vi "TX_POWER(DEBUG).vi"() -> ()   [LabVIEW 2015]
uses:
  <instrlib>/Rohde&Schwarz Spectrum Analyzer/Rohde&Schwarz Spectrum Analyzer.lvlib
panel:
  in  "O_R&S Spec1 2":refnum<visa-resource-name>
  in  "O_R&S Spec1":refnum<visa-resource-name>="GPIB0::22::INSTR"
  out "R_B_peak":dbl[](array[numeric])
  out "R_B_pos":dbl[](array[numeric])
  out "R_A_peak":dbl[](array[numeric])
  out "R_A_pos":dbl[](array[numeric])
  out "B通道接收带":cluster{"X":dbl[], "Amplitude":dbl[]}(graph)
  out "B通道发射带":cluster{"X":dbl[], "Amplitude":dbl[]}(graph)
  out "A通道发射带":cluster{"X":dbl[], "Amplitude":dbl[]}(graph)
  out "A通道接收带":cluster{"X":dbl[], "Amplitude":dbl[]}(graph)
  in  "接收带末频率(Mhz)":u32=2300 caption="Start Frequency (0.0)"
  in  "接收带始频率(Mhz)":u32=2200 caption="Stop Frequency (0.0)"
  out "R_B_paek":dbl caption="Marker Amplitude" format="%^.3e"
  out "R_B_pos":dbl caption="Marker Position" format="%^.3e"
  out "Amplitude 2":dbl[](array[numeric]) caption="Amplitude" format="%^.3e"
  out "X 2":dbl[](array[numeric]) caption="X" format="%^.3e"
  out "R_A_peak":dbl caption="Marker Amplitude" format="%^.3e"
  out "R_A_pos":dbl caption="Marker Position" format="%^.3e"
  out "Amplitude":dbl[](array[numeric]) format="%^.3e"
  out "X":dbl[](array[numeric]) format="%^.3e"
  in  "发射带末频率(Mhz)":u32=2130 caption="Start Frequency (0.0)"
  in  "发射带始频率(Mhz)":u32=2018 caption="Stop Frequency (0.0)"
  out "B_peak":dbl[](array[numeric])
  out "B_pos":dbl[](array[numeric])
  out "B_next_pos":dbl[](array[numeric])
  out "B_peak_next":dbl[](array[numeric])
  out "Array 6":cluster{"X":dbl[], "Amplitude":dbl[]}[](array[cluster])
  out "A_peak":dbl[](array[numeric])
  out "A_pos":dbl[](array[numeric])
  out "A_next_pos":dbl[](array[numeric])
  out "A_peak_next":dbl[](array[numeric])
  out "Array":cluster{"X":dbl[], "Amplitude":dbl[]}[](array[cluster])
  in  "OK":bool
  in  "stop":bool
  out "Bx":dbl[](array[numeric]) caption="X" format="%^.3e"
  out "By":dbl[](array[numeric]) caption="Amplitude" format="%^.3e"
  out "B_pos":dbl caption="Marker Position" format="%^.3e"
  out "B_peak":dbl caption="Marker Amplitude" format="%^.3e"
  out "B_next_pos":dbl caption="Marker Position" format="%^.3e"
  out "B_peak_next":dbl caption="Marker Amplitude" format="%^.3e"
  out "A_peak_next":dbl caption="Marker Amplitude" format="%^.3e"
  out "A_next_pos":dbl caption="Marker Position" format="%^.3e"
  out "A_peak":dbl caption="Marker Amplitude" format="%^.3e"
  out "A_pos":dbl caption="Marker Position" format="%^.3e"
  out "Ay":dbl[](array[numeric]) caption="Amplitude" format="%^.3e"
  out "Ax":dbl[](array[numeric]) caption="X" format="%^.3e"
  in  "VISA resource name 2":refnum<visa-resource-name>="COM3"
  out "Freq_Tab":u32[](array[numeric])
  in  "Insert Point":u32
  in  "EABLE Insert":bool
  in  "Value":u32=10 caption="Point Num"
  in  "cnt/setp":enum16{"SETP", "COUNT"}(ring)=enum."COUNT"
  in  "freq_max(Mhz)":u32=2123
  in  "freq_min(Mhz)":u32=2018
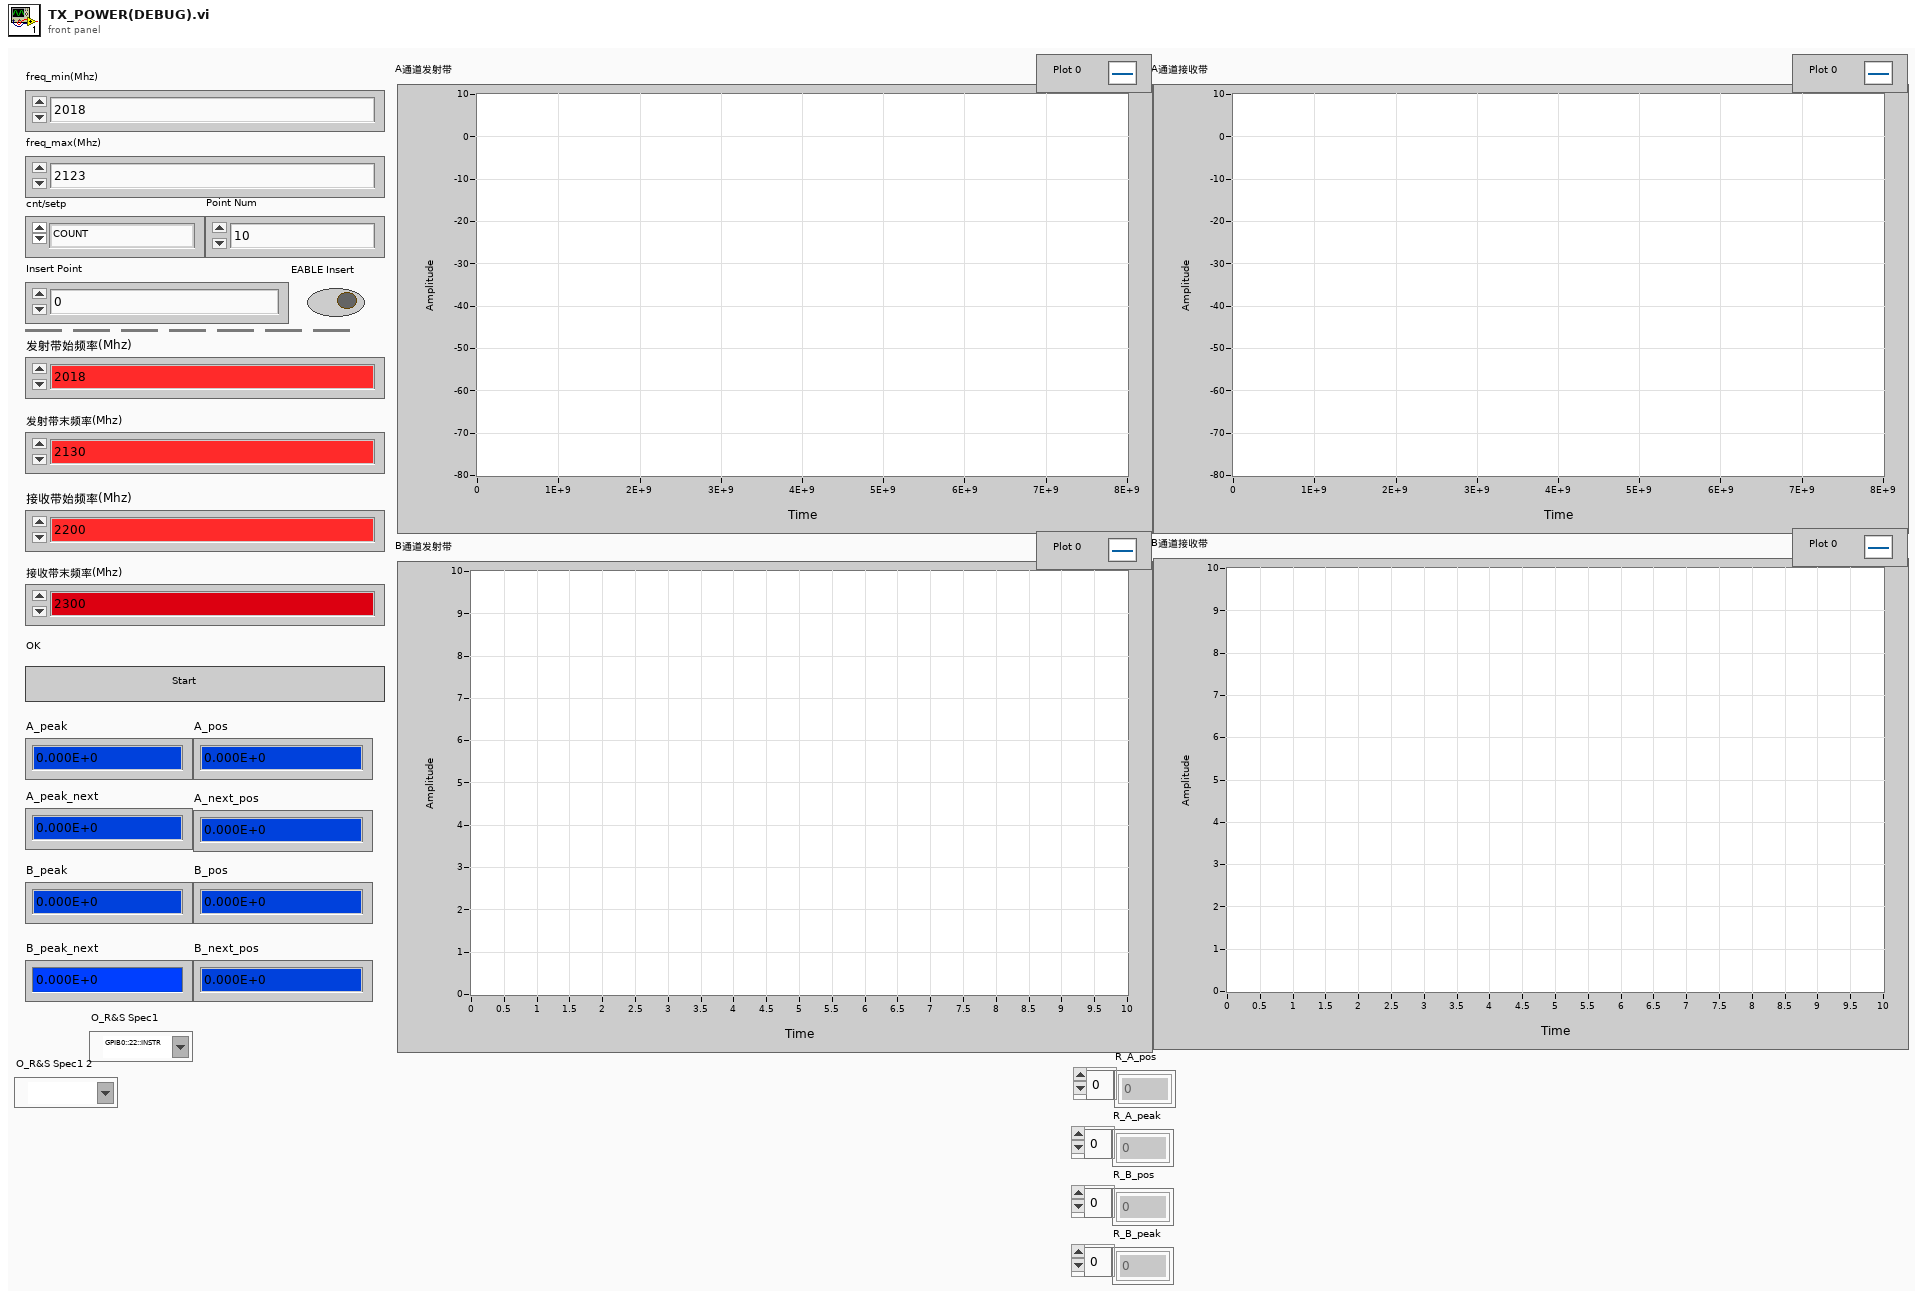
[diagram p1: front panel]
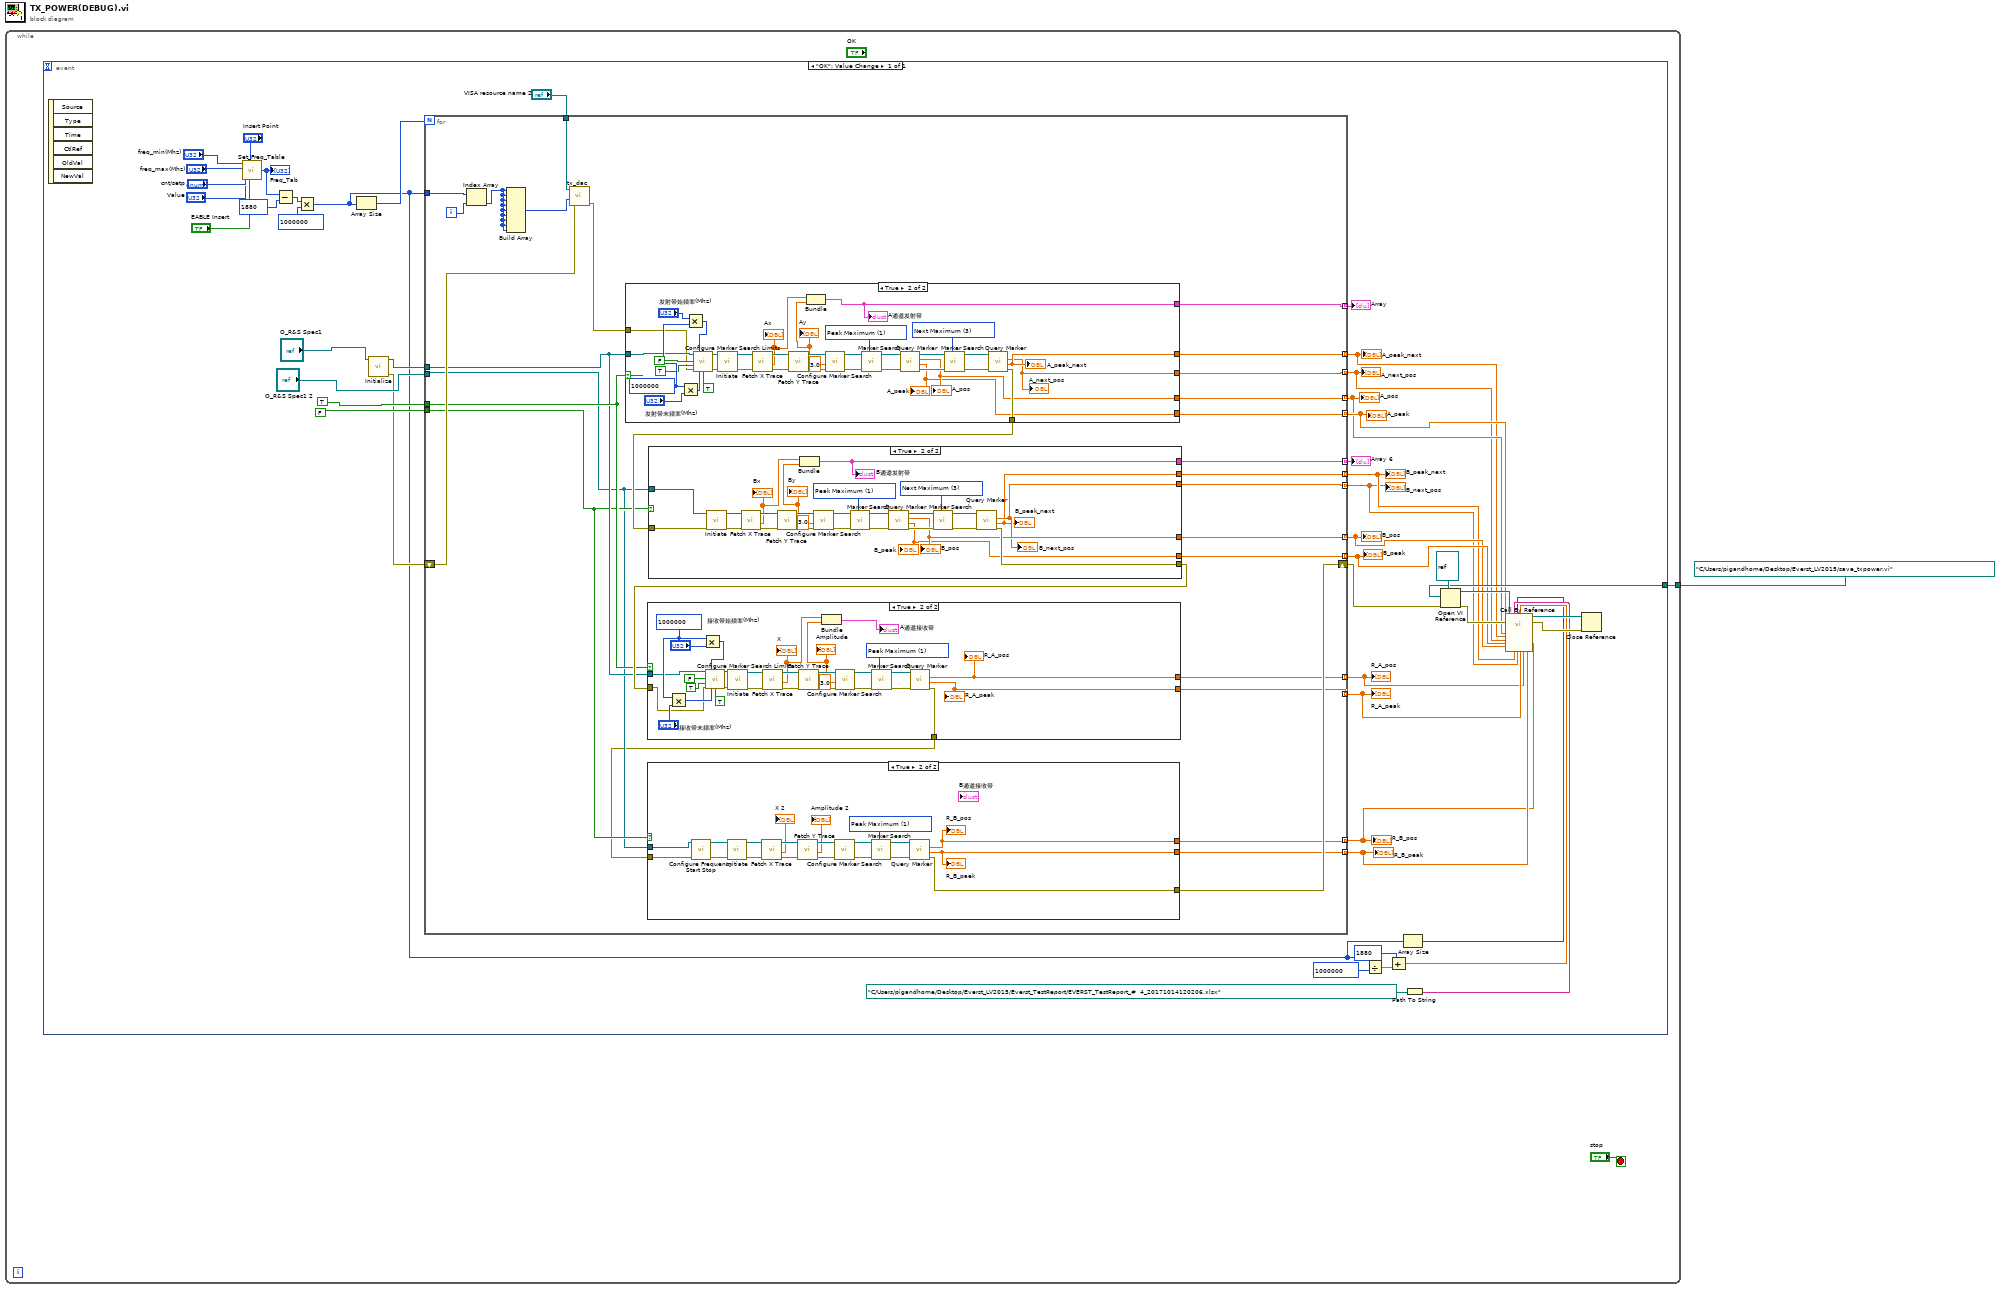
[diagram p0: block diagram]
diagram:
  n1 = while {
    tunnel: path "C:/Users/pigandhome/Desktop/Everst_LV2015/save_txpower.vi" ("vi path") -> [w2]
    stop <- "stop" stop-if-true
    n2 = event shown="[0] \"OK\": Value Change" {
      selector: _ -> [_]
      dyn-events: _ -> [_]
      timeout: _ -> [_]
      tunnel: w2 -> [w30]
      event "OK": Value Change {
        n3 = event-data() -> ()  [unwired: 1 in, 6 out]
        n4 = call "Set_Freq_Table.vi"("EABLE Insert"="EABLE Insert", "Insert Point"="Insert Point", "Value"="Value", "cnt/setp"="cnt/setp", "freq_max(Mhz)"="freq_max(Mhz)", "freq_min(Mhz)"="freq_min(Mhz)") -> ("Freq_Tab"=w44:u32[])
        "Freq_Tab" <- w44
        n5 = Subtract(x=w44, y=1880) -> (x-y=w42:u32[])
        n6 = Multiply(x=w42, y=1000000) -> (x*y=w5:u32[])
        n7 = Array Size(array=w5) -> (size(s)=w40:i32)
        n8 = call <instrlib>:"Initialize.vi"("VISA resource name"="O_R&S Spec1") -> ("VISA resource name out"=w24:refnum<visa-resource-name>, "error out"=w22:errorcluster)  [unwired: 13 in]
        n9 = for {
          N: w40 -> [_]
          tunnel: w5 -> [w78]
          tunnel: "VISA resource name 2" -> [w77]
          tunnel: w24 -> [w59]
          tunnel: "O_R&S Spec1 2" -> [w57]
          tunnel: TRUE ("spec1_state") -> [w60]
          tunnel: FALSE ("spec1_state") -> [w58]
          shift-right: [w55] -> w31
          shift-left: w22 -> [w73]
          tunnel: [w71] -> w15 mode=indexing
          tunnel: [w70] -> w14 mode=indexing
          tunnel: [w69] -> w16 mode=indexing
          tunnel: [w68] -> w17 mode=indexing
          tunnel: [w67] -> w10 mode=indexing
          tunnel: [w66] -> w11 mode=indexing
          tunnel: [w65] -> w12 mode=indexing
          tunnel: [w64] -> w13 mode=indexing
          tunnel: [w63] -> w38 mode=indexing
          tunnel: [w62] -> w37 mode=indexing
          tunnel: [w54] -> w8 mode=indexing
          tunnel: [w53] -> w9 mode=indexing
          tunnel: [w52] -> w6 mode=indexing
          tunnel: [w51] -> w7 mode=indexing
          i -> [w79]
          n10 = Index Array(array=w78, index=w79) -> (element=w72:u32)
          n11 = Build Array(w72, w72, w72, w72, w72, w72, w72, w72, w72) -> (w76:u32[])
          n12 = call "tx_dac.vi"("error in (no error)"=w73, "fin"=w76, "VISA resource name 2"=w77) -> ("error out"=w75:errorcluster)  [unwired: 3 in]
          n13 = case shown="True" w60 {
            tunnel: w59 -> [_ w164]
            tunnel: w75 -> [w160 w163]
            tunnel: [w160 w180] -> w74
            tunnel: [_ w162] -> w71
            tunnel: [_ w161] -> w70
            tunnel: [_ w179] -> w69
            tunnel: [_ w178] -> w68
            tunnel: [_ w172] -> w63
            frame False {
            }
            frame True {
              w173 = u32 1000000 ("x")
              w181 = 3 items=["Peak Maximum"=1, "Peak Minimum"=2, "Next Maximum"=3, "Left Maximum"=4, "Right Maximum"=5, "Next Minimum"=6, "Left Minimum"=7, "Right Minimum"=8] ("Marker Search (Peak Maximum)")
              w182 = 1 items=["Peak Maximum"=1, "Peak Minimum"=2, "Next Maximum"=3, "Left Maximum"=4, "Right Maximum"=5, "Next Minimum"=6, "Left Minimum"=7, "Right Minimum"=8] ("Marker Search (Peak Maximum)")
              n14 = Multiply(x=w173, y="发射带末频率(Mhz)") -> (x*y=w168:u32)
              n15 = Multiply(x="发射带始频率(Mhz)", y=w173) -> (x*y=w169:u32)
              n16 = call <instrlib>:"Configure Marker Search Limits.vi"("VISA resource name"=w164, "Search Limit Left (0.0)"=w169, "Threshold State (T: On)"=FALSE, "Search Limits (F: Off)"=TRUE, "error in (no error)"=w163, "Search Limit Right (0.0)"=w168, "Search Limits Zoom (F: Off)"=TRUE) -> ("VISA resource name out"=w170:refnum<visa-resource-name>, "error out"=w171:errorcluster)  [unwired: 7 in]
              n17 = call <instrlib>:"Initiate.vi"("error in (no error)"=w171, "VISA resource name"=w170) -> ("error out"=w197:errorcluster, "VISA resource name out"=w196:refnum<visa-resource-name>)  [unwired: 8 in]
              n18 = call <instrlib>:"Fetch X Trace.vi"("error in (no error)"=w197, "VISA resource name"=w196) -> ("error out"=w195:errorcluster, "X"=w177:dbl[], "VISA resource name out"=w194:refnum<visa-resource-name>)  [unwired: 7 in]
              "Ax" <- w177
              n19 = call <instrlib>:"Fetch Y Trace.vi"("error in (no error)"=w195, "VISA resource name"=w194) -> ("error out"=w193:errorcluster, "Amplitude"=w176:dbl[], "VISA resource name out"=w192:refnum<visa-resource-name>)  [unwired: 7 in]
              "Ay" <- w176
              n20 = Bundle("X"=w177, "Amplitude"=w176) -> (w172:cluster{"X":dbl[], "Amplitude":dbl[]})  [unwired: 1 in]
              "A通道发射带" <- w172
              n21 = call <instrlib>:"Configure Marker Search.vi"("error in (no error)"=w193, "Peak Excursion (6.0)"=3.0, "VISA resource name"=w192) -> ("error out"=w191:errorcluster, "VISA resource name out"=w190:refnum<visa-resource-name>)  [unwired: 7 in]
              n22 = call <instrlib>:"Marker Search.vi"("Marker Search (Peak Maximum)"=w182, "error in (no error)"=w191, "VISA resource name"=w190) -> ("error out"=w189:errorcluster, "VISA resource name out"=w188:refnum<visa-resource-name>)  [unwired: 7 in]
              n23 = call <instrlib>:"Query Marker.vi"("error in (no error)"=w189, "VISA resource name"=w188) -> ("error out"=w187:errorcluster, "Marker Amplitude"=w178:dbl, "Marker Position"=w179:dbl, "VISA resource name out"=w186:refnum<visa-resource-name>)  [unwired: 6 in]
              "A_pos" <- w179
              "A_peak" <- w178
              n24 = call <instrlib>:"Marker Search.vi"("Marker Search (Peak Maximum)"=w181, "error in (no error)"=w187, "VISA resource name"=w186) -> ("error out"=w185:errorcluster, "VISA resource name out"=w184:refnum<visa-resource-name>)  [unwired: 7 in]
              n25 = call <instrlib>:"Query Marker.vi"("error in (no error)"=w185, "VISA resource name"=w184) -> ("error out"=w180:errorcluster, "Marker Amplitude"=w162:dbl, "Marker Position"=w161:dbl)  [unwired: 6 in, 1 out]
              "A_next_pos" <- w161
              "A_peak_next" <- w162
            }
          }
          n26 = case shown="True" w58 {
            tunnel: w57 -> [_ w142]
            tunnel: w74 -> [w132 w141]
            tunnel: [w132 w140] -> w61
            tunnel: [_ w134] -> w67
            tunnel: [_ w133] -> w66
            tunnel: [_ w139] -> w65
            tunnel: [_ w138] -> w64
            tunnel: [_ w135] -> w62
            frame False {
            }
            frame True {
              w159 = 3 items=["Peak Maximum"=1, "Peak Minimum"=2, "Next Maximum"=3, "Left Maximum"=4, "Right Maximum"=5, "Next Minimum"=6, "Left Minimum"=7, "Right Minimum"=8] ("Marker Search (Peak Maximum)")
              w158 = 1 items=["Peak Maximum"=1, "Peak Minimum"=2, "Next Maximum"=3, "Left Maximum"=4, "Right Maximum"=5, "Next Minimum"=6, "Left Minimum"=7, "Right Minimum"=8] ("Marker Search (Peak Maximum)")
              n27 = call <instrlib>:"Initiate.vi"("error in (no error)"=w141, "VISA resource name"=w142) -> ("error out"=w143:errorcluster, "VISA resource name out"=w144:refnum<visa-resource-name>)  [unwired: 8 in]
              n28 = call <instrlib>:"Fetch X Trace.vi"("error in (no error)"=w143, "VISA resource name"=w144) -> ("error out"=w145:errorcluster, "X"=w137:dbl[], "VISA resource name out"=w146:refnum<visa-resource-name>)  [unwired: 7 in]
              "Bx" <- w137
              n29 = call <instrlib>:"Fetch Y Trace.vi"("error in (no error)"=w145, "VISA resource name"=w146) -> ("error out"=w147:errorcluster, "Amplitude"=w136:dbl[], "VISA resource name out"=w148:refnum<visa-resource-name>)  [unwired: 7 in]
              "By" <- w136
              n30 = Bundle("X"=w137, "Amplitude"=w136) -> (w135:cluster{"X":dbl[], "Amplitude":dbl[]})  [unwired: 1 in]
              "B通道发射带" <- w135
              n31 = call <instrlib>:"Configure Marker Search.vi"("error in (no error)"=w147, "Peak Excursion (6.0)"=3.0, "VISA resource name"=w148) -> ("error out"=w149:errorcluster, "VISA resource name out"=w150:refnum<visa-resource-name>)  [unwired: 7 in]
              n32 = call <instrlib>:"Marker Search.vi"("Marker Search (Peak Maximum)"=w158, "error in (no error)"=w149, "VISA resource name"=w150) -> ("error out"=w151:errorcluster, "VISA resource name out"=w152:refnum<visa-resource-name>)  [unwired: 7 in]
              n33 = call <instrlib>:"Query Marker.vi"("error in (no error)"=w151, "VISA resource name"=w152) -> ("error out"=w153:errorcluster, "Marker Amplitude"=w138:dbl, "Marker Position"=w139:dbl, "VISA resource name out"=w154:refnum<visa-resource-name>)  [unwired: 6 in]
              "B_pos" <- w139
              "B_peak" <- w138
              n34 = call <instrlib>:"Marker Search.vi"("Marker Search (Peak Maximum)"=w159, "error in (no error)"=w153, "VISA resource name"=w154) -> ("error out"=w155:errorcluster, "VISA resource name out"=w156:refnum<visa-resource-name>)  [unwired: 7 in]
              n35 = call <instrlib>:"Query Marker.vi"("error in (no error)"=w155, "VISA resource name"=w156) -> ("error out"=w140:errorcluster, "Marker Amplitude"=w133:dbl, "Marker Position"=w134:dbl)  [unwired: 6 in, 1 out]
              "B_next_pos" <- w134
              "B_peak_next" <- w133
            }
          }
          n36 = case shown="True" w60 {
            tunnel: w61 -> [w101 w104]
            tunnel: w59 -> [_ w105]
            tunnel: [w101 w117] -> w56
            tunnel: [_ w103] -> w54
            tunnel: [_ w102] -> w53
            frame False {
            }
            frame True {
              w114 = u32 1000000
              w120 = 1 items=["Peak Maximum"=1, "Peak Minimum"=2, "Next Maximum"=3, "Left Maximum"=4, "Right Maximum"=5, "Next Minimum"=6, "Left Minimum"=7, "Right Minimum"=8] ("Marker Search (Peak Maximum)")
              n37 = Multiply(x=w114, y="接收带末频率(Mhz)") -> (x*y=w109:u32)
              n38 = Multiply(x=w114, y="接收带始频率(Mhz)") -> (x*y=w110:u32)
              n39 = call <instrlib>:"Configure Marker Search Limits.vi"("VISA resource name"=w105, "Search Limit Left (0.0)"=w110, "Threshold State (T: On)"=FALSE, "Search Limits (F: Off)"=TRUE, "error in (no error)"=w104, "Search Limit Right (0.0)"=w109, "Search Limits Zoom (F: Off)"=TRUE) -> ("VISA resource name out"=w112:refnum<visa-resource-name>, "error out"=w111:errorcluster)  [unwired: 7 in]
              n40 = call <instrlib>:"Initiate.vi"("error in (no error)"=w111, "VISA resource name"=w112) -> ("error out"=w131:errorcluster, "VISA resource name out"=w126:refnum<visa-resource-name>)  [unwired: 8 in]
              n41 = call <instrlib>:"Fetch X Trace.vi"("error in (no error)"=w131, "VISA resource name"=w126) -> ("error out"=w130:errorcluster, "X"=w119:dbl[], "VISA resource name out"=w125:refnum<visa-resource-name>)  [unwired: 7 in]
              "X" <- w119
              n42 = call <instrlib>:"Fetch Y Trace.vi"("error in (no error)"=w130, "VISA resource name"=w125) -> ("error out"=w129:errorcluster, "Amplitude"=w118:dbl[], "VISA resource name out"=w124:refnum<visa-resource-name>)  [unwired: 7 in]
              "Amplitude" <- w118
              n43 = Bundle("X"=w119, "Amplitude"=w118) -> (→"A通道接收带":cluster{"X":dbl[], "Amplitude":dbl[]})  [unwired: 1 in]
              n44 = call <instrlib>:"Configure Marker Search.vi"("error in (no error)"=w129, "Peak Excursion (6.0)"=3.0, "VISA resource name"=w124) -> ("error out"=w128:errorcluster, "VISA resource name out"=w123:refnum<visa-resource-name>)  [unwired: 7 in]
              n45 = call <instrlib>:"Marker Search.vi"("Marker Search (Peak Maximum)"=w120, "error in (no error)"=w128, "VISA resource name"=w123) -> ("error out"=w127:errorcluster, "VISA resource name out"=w122:refnum<visa-resource-name>)  [unwired: 7 in]
              n46 = call <instrlib>:"Query Marker.vi"("error in (no error)"=w127, "VISA resource name"=w122) -> ("error out"=w117:errorcluster, "Marker Amplitude"=w102:dbl, "Marker Position"=w103:dbl)  [unwired: 6 in, 1 out]
              "R_A_pos" <- w103
              "R_A_peak" <- w102
            }
          }
          n47 = case shown="True" w58 {
            tunnel: w57 -> [_ w85]
            tunnel: w56 -> [w80 w84]
            tunnel: [w80 w83] -> w55
            tunnel: [_ w82] -> w52
            tunnel: [_ w81] -> w51
            frame False {
            }
            frame True {
              w86 = 1 items=["Peak Maximum"=1, "Peak Minimum"=2, "Next Maximum"=3, "Left Maximum"=4, "Right Maximum"=5, "Next Minimum"=6, "Left Minimum"=7, "Right Minimum"=8] ("Marker Search (Peak Maximum)")
              n48 = call <instrlib>:"Configure Frequency Start Stop.vi"("error in (no error)"=w84, "VISA resource name"=w85) -> ("error out"=w100:errorcluster, "VISA resource name out"=w99:refnum<visa-resource-name>)  [unwired: 8 in]
              n49 = call <instrlib>:"Initiate.vi"("error in (no error)"=w100, "VISA resource name"=w99) -> ("error out"=w98:errorcluster, "VISA resource name out"=w97:refnum<visa-resource-name>)  [unwired: 8 in]
              n50 = call <instrlib>:"Fetch X Trace.vi"("error in (no error)"=w98, "VISA resource name"=w97) -> ("error out"=w96:errorcluster, "X"=→"X 2":dbl[], "VISA resource name out"=w95:refnum<visa-resource-name>)  [unwired: 7 in]
              n51 = call <instrlib>:"Fetch Y Trace.vi"("error in (no error)"=w96, "VISA resource name"=w95) -> ("error out"=w94:errorcluster, "Amplitude"=→"Amplitude 2":dbl[], "VISA resource name out"=w93:refnum<visa-resource-name>)  [unwired: 7 in]
              n52 = call <instrlib>:"Configure Marker Search.vi"("error in (no error)"=w94, "VISA resource name"=w93) -> ("error out"=w92:errorcluster, "VISA resource name out"=w91:refnum<visa-resource-name>)  [unwired: 8 in]
              n53 = call <instrlib>:"Marker Search.vi"("Marker Search (Peak Maximum)"=w86, "error in (no error)"=w92, "VISA resource name"=w91) -> ("error out"=w90:errorcluster, "VISA resource name out"=w89:refnum<visa-resource-name>)  [unwired: 7 in]
              n54 = call <instrlib>:"Query Marker.vi"("error in (no error)"=w90, "VISA resource name"=w89) -> ("error out"=w83:errorcluster, "Marker Amplitude"=w81:dbl, "Marker Position"=w82:dbl)  [unwired: 6 in, 1 out]
              "R_B_pos" <- w82
              "R_B_paek" <- w81
            }
          }
        }
        "Array" <- w38
        "A_peak_next" <- w15
        "A_next_pos" <- w14
        "A_pos" <- w16
        "A_peak" <- w17
        "Array 6" <- w37
        "B_peak_next" <- w11
        "B_next_pos" <- w10
        "B_pos" <- w12
        "B_peak" <- w13
        "R_A_pos" <- w8
        "R_A_peak" <- w9
        "R_B_pos" <- w6
        "R_B_peak" <- w7
        n55 = Divide(x=w5, y=u32 1000000) -> (x/y=w20:dbl[])
        n56 = Add(x=u32 1880, y=w20) -> (x+y=w18:dbl[])
        n57 = Array Size(array=w5) -> (size(s)=w4:i32)
        n58 = Path To String(path=path "C:/Users/pigandhome/Desktop/Everst_LV2015/Everst_TestReport/EVERST_TestReport_#  4_20171014120206.xlsx") -> (string=w29:string)
        n59 = Open VI Reference(type specifier VI Refnum (for type only)=refnum<vi> refnum, vi path=w30, error in (no error)=w31) -> (vi reference=w36:refnum<vi>, error out=w35:errorcluster)  [unwired: 3 in]
        n60 = call-by-ref "?"(reference=w36, error in=w35, "Apeak"=w17, "Apeakpos"=w16, "Apeaknext"=w15, "Anextpos"=w14, "Bpeak"=w13, "Bpeakpos"=w12, "PATH"=w29, "Bpeaknext"=w11, "Tabsize"=w4, "Bnextpos"=w10, "FreqTab"=w18, "RApeak"=w9, "RApos"=w8, "RBpos"=w6, "RBpeak"=w7) -> (reference out=w32:refnum<vi>, error out=w33:errorcluster)  [unwired: 5 in]
        n61 = Close Reference(reference=w32, error in (no error)=w33) -> ()  [unwired: 1 out]
      }
    }
  }
